vi "VerifConfigState.vi"(8 "error in (no error)":errorcluster, 11 "S4GUI in":refnum<class "S4GUI.lvclass">) -> (0 "error out":errorcluster, 3 "S4GUI out":refnum<class "S4GUI.lvclass">)   [LabVIEW 2018, in "S4GUI.lvclass"]
uses:
  S4GUI/S4GUI.lvclass
  S4GUI/S4GUI.lvclass/S4GUI.ctl
  Acquisition/Acquisition.lvclass
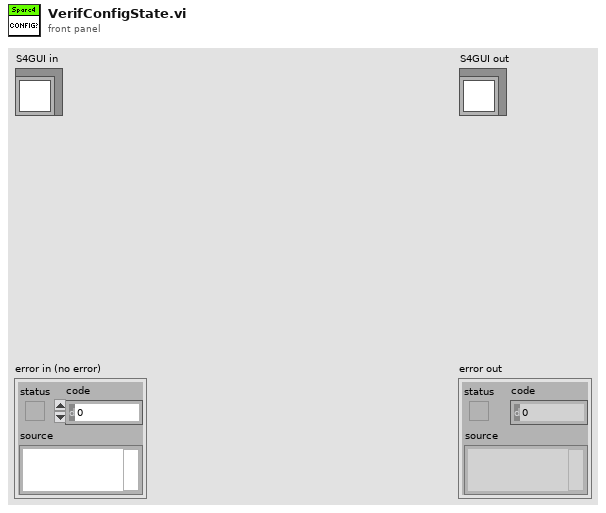
[diagram p1: front panel]
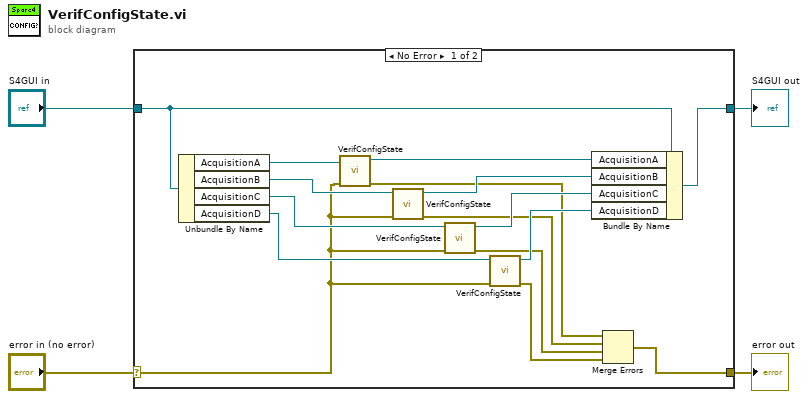
[diagram p0: block diagram]
diagram:
  n1 = case shown="No Error" "error in (no error)" {
    selector: "error in (no error)" -> [w10 w22]
    tunnel: [w5 w22] -> w3
    tunnel: [w15 w21] -> w1
    tunnel: "S4GUI in" -> [w16 w21]
    frame No Error {
      n2 = Unbundle By Name(w16) -> ("AcquisitionA"=w20:refnum<class "Acquisition.lvclass">, "AcquisitionB"=w19:refnum<class "Acquisition.lvclass">, "AcquisitionC"=w18:refnum<class "Acquisition.lvclass">, "AcquisitionD"=w17:refnum<class "Acquisition.lvclass">)
      n3 = call-dynamic "VerifConfigState.vi"("error in (no error)"=w10, "Acquisition in"=w20) -> ("error out"=w9:errorcluster, "Acquisition out"=w14:refnum<class "Acquisition.lvclass">)  [unwired: 8 in]
      n4 = call-dynamic "VerifConfigState.vi"("error in (no error)"=w10, "Acquisition in"=w19) -> ("error out"=w8:errorcluster, "Acquisition out"=w13:refnum<class "Acquisition.lvclass">)  [unwired: 8 in]
      n5 = call-dynamic "VerifConfigState.vi"("error in (no error)"=w10, "Acquisition in"=w18) -> ("error out"=w7:errorcluster, "Acquisition out"=w12:refnum<class "Acquisition.lvclass">)  [unwired: 8 in]
      n6 = call-dynamic "VerifConfigState.vi"("error in (no error)"=w10, "Acquisition in"=w17) -> ("error out"=w6:errorcluster, "Acquisition out"=w11:refnum<class "Acquisition.lvclass">)  [unwired: 8 in]
      n7 = Bundle By Name(cluster=w16, "AcquisitionA"=w14, "AcquisitionB"=w13, "AcquisitionC"=w12, "AcquisitionD"=w11) -> (w15:refnum<class "S4GUI.lvclass">)
      n8 = Merge Errors(w9, w8, w7, w6) -> (w5:errorcluster)
    }
    frame Error {
    }
  }
  "error out" <- w3
  "S4GUI out" <- w1
